vi "TestInitializeLocalLog_InjectEditTimeAbsRunTimeConcrete_LogEventCaptured.vi"(8 "error in (no error)":errorcluster, 11 "TestCase in":refnum<class "TestMalleableInterface.lvclass">) -> (0 "error out":errorcluster, 3 "TestCase out":refnum<class "TestMalleableInterface.lvclass">)   [LabVIEW 2017, in "TestMalleableInterface.lvclass"]
uses:
  TestMalleableInterface.lvclass
  Source/Composed Log/Log Sink/Log Sink.lvclass
  Source/LVQueue Sink/LVQueue Sink.lvclass/LVQueue Sink.ctl
  Source/Composed Log/LoggerReference/LoggerReference.lvclass/LoggerReference.ctl
  8d299841-f253-422a-a7a1-59edf70c310f.vi
  Source/Composed Log/LoggerReference/Return Aggregate Queues.vi
  Source/Composed Log/LoggerReference/Add Aggregate Log.vi
  8d299841-f253-422a-a7a1-59edf70c310f.vi/6ab769d7-668d-47b9-a7ef-c2c22b3e353b.vi
  Source/Composed Log/LoggerReference/Log.vi
  Source/Composed Log/LoggerReference/Send Add Sink.vi
  Source/Composed Log/LoggerReference/Remove Stale Logs.vi
  Source/LVQueue Sink/LVQueue Sink.lvclass
  C:/CS/Internal/LabVIEW/Logger/Source/Composed Log/Log Sink/Log Sink.lvclass
  Source/Composed Log/Application Logger/Launch Worker Loop.vi
  Source/Composed Log/LoggerReference/Initialize Logger Instance.vi
  Source/Composed Log/LoggerReference/LoggerReference.lvclass
  Source/Composed Log/IErrorFormat/IErrorFormat.lvclass
  <vilib>/addons/_JKI Toolkits/VI Tester/TestCase.llb/TestCase.lvclass
  C:/Program Files (x86)/National Instruments/LabVIEW 2017/vi.lib/addons/_JKI Toolkits/VI Tester/TestCase.llb/TestCase.lvclass
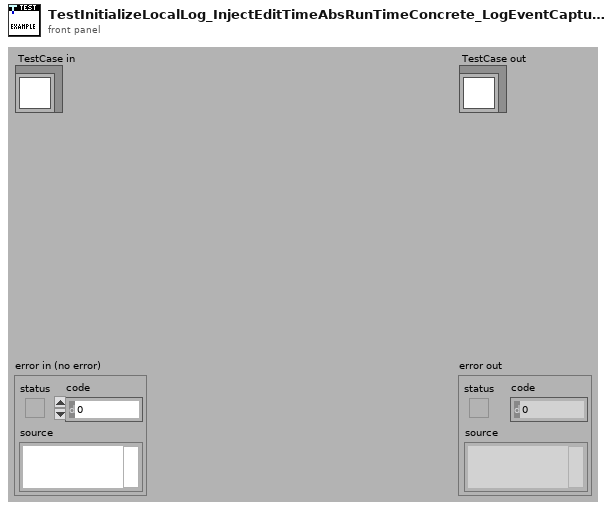
[diagram p1: front panel]
types:
  T1 = typedef "Composed Log.lvlib/Log Packet.ctl" = cluster{"Data To Log":string, "Source":string, "Event Level":T2, "Event Time":timestamp}
  T2 = typedef "Composed Log.lvlib/Log Level.ctl" = enum16{"Debug", "Info", "Warning", "Error", "Critical"}
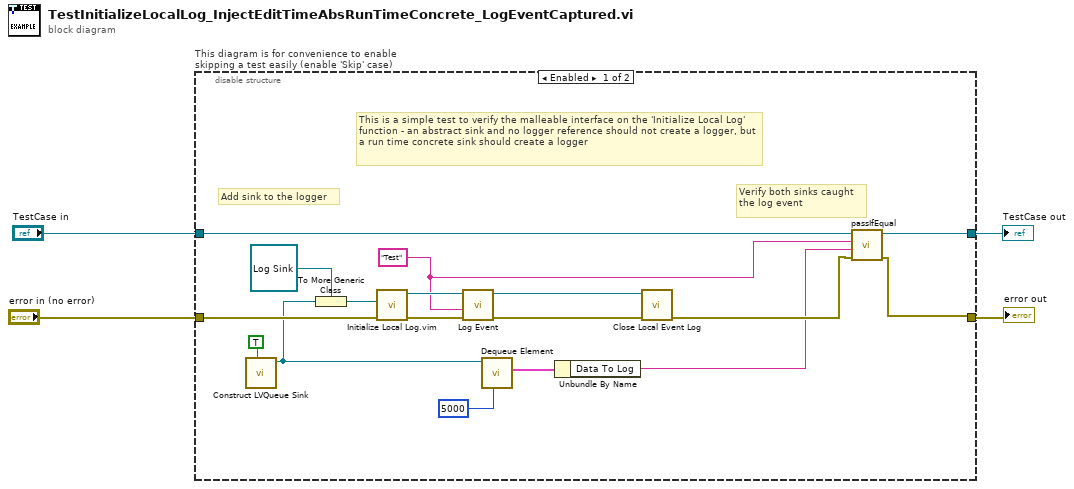
[diagram p0: block diagram]
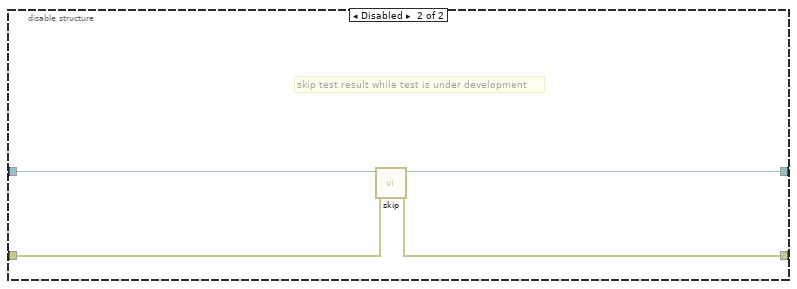
[diagram p2: hidden frame]
diagram:
  n1 = disable-structure "This diagram is for convenience to enable skipping a test easily (enable 'Skip' case)" shown="Enabled" {
    disable-tunnel: "TestCase in" -> [w12 w25]
    disable-tunnel: [w11 w23] -> w1
    disable-tunnel: [w13 w24] -> w3
    disable-tunnel: "error in (no error)" -> [w8 w22]
    frame Enabled {
      w9 = "Test" ("SourceID")
      # "This is a simple test to verify the malleable interface on the 'Initialize Local Log' function - an abstract sink and no logger reference should not create a logger, but a run time concrete sink should create a logger"
      # "Verify both sinks caught the log event"
      # "Add sink to the logger"
      n2 = call "Construct LVQueue Sink.vi"("User Shutdown? (F)"=TRUE) -> ("LVQueue Sink out"=w7:refnum<class "LVQueue Sink.lvclass">)  [unwired: 9 in, 1 out]
      n3 = To More Generic Class(target class=refnum<class "Log Sink.lvclass"> refnum ("Startup Sink(s)"), reference=w7) -> (generic class reference=w6:refnum<class "Log Sink.lvclass">)
      n4 = call "Initialize Local Log.vim"("error in (no error)"=w8, "Startup Sink(s)"=w6) -> ("error out"=w17:errorcluster, "Log Instance Reference"=w18:refnum<class "LoggerReference.lvclass">)  [unwired: 7 in, 1 out]
      n5 = call "Log Event.vi"("error in (no error)"=w17, "Data To Log"=w9, "Log Instance"=w18) -> ("error out"=w20:errorcluster, "Log Instance Out"=w19:refnum<class "LoggerReference.lvclass">)  [unwired: 7 in]
      n6 = call "Dequeue Element.vi"("timeout in ms (-1)"=5000, "LVQueue Sink in"=w7) -> ("Log Packet"=w16:T1)  [unwired: 6 in, 3 out]
      n7 = Unbundle By Name(w16) -> ("Data To Log"=w10:string)
      n8 = call "Close Local Event Log.vi"("error in (no error)"=w20, "Log Instance"=w19) -> ("error out"=w14:errorcluster)  [unwired: 9 in]
      n9 = call-dynamic "passIfEqual.vi"("error in (no error)"=w14, "y"=w10, "x"=w9, "TestCase in"=w12) -> ("error out"=w13:errorcluster, "TestCase out"=w11:refnum<class "TestMalleableInterface.lvclass">)  [unwired: 6 in]
    }
    frame Disabled {
      # "skip test result while test is under development"
      n10 = call <vilib>:"skip.vi"("error in (no error)"=w22, "TestCase in"=w25) -> ("error out"=w24:errorcluster, "TestCase out"=w23:refnum<class "TestMalleableInterface.lvclass">)  [unwired: 8 in]
    }
  }
  "error out" <- w3
  "TestCase out" <- w1
